vi "Create.vi"(8 "error in (no error)":errorcluster, 11 "String array in":string[](array[string])) -> (0 "error out":errorcluster, 3 "StringArray out":refnum<class "StringArray.lvclass">)   [LabVIEW 2012, in "MDSplus.lvlib" / "StringArray.lvclass"]
uses:
  <vilib>/MDSplus/Classes/Data_Class/Array_Class/StringArray_Class/StringArray.lvclass
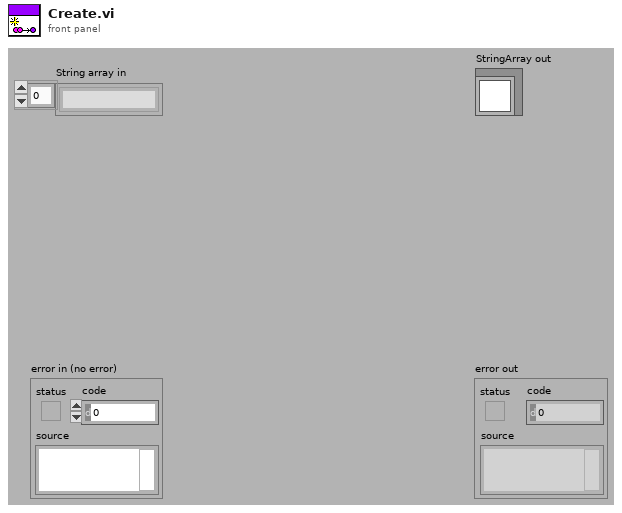
[diagram p1: front panel]
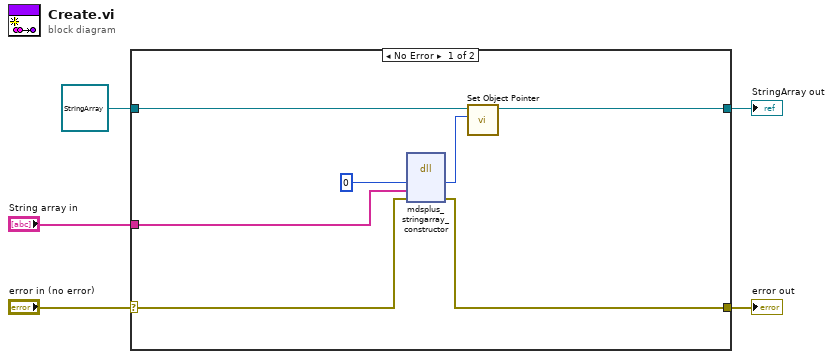
[diagram p0: block diagram]
diagram:
  n1 = case shown="No Error" "error in (no error)" {
    selector: "error in (no error)" -> [w10 w14]
    tunnel: [w6 w14] -> w4
    tunnel: [w8 w13] -> w2
    tunnel: refnum<class "StringArray.lvclass"> refnum ("Float32 in") -> [w9 w13]
    tunnel: "String array in" -> [w7 _]
    frame No Error {
      n2 = dll-call lib="MDSobjectsLVShr" fn="mdsplus_stringarray_constructor"("lvStringArrayPtrOut"=i64 0 ("lvTreePtr"), "lvLStrArrHdlIn"=w7, "error"=w10) -> ("lvStringArrayPtrOut"=w11:i64, "error"=w6:errorcluster)  [unwired: 5 in, 2 out]
      n3 = call-dynamic "Set Object Pointer.vi"("Object Pointer"=w11, "Data in"=w9) -> ("Data out"=w8:refnum<class "StringArray.lvclass">)  [unwired: 9 in]
    }
    frame Error {
    }
  }
  "error out" <- w4
  "StringArray out" <- w2
